vi "Test Step Stability.vi"(8 "Ranges":dbl[](array[numeric]), 9 "Setpoints":dbl[](array[numeric]), 11 "Array":refnum<class "TimeBasedQueue.lvclass">[](array[class])) -> (0 "Min":dbl[](array[numeric]), 1 "Components Stable?":bool[](array[boolean]), 2 "Max":dbl[](array[numeric]), 3 "System Stable?":bool)   [LabVIEW 2012, in "TimeBasedQueue.lvclass"]
uses:
  Time Based Queue/TimeBasedQueue.lvclass
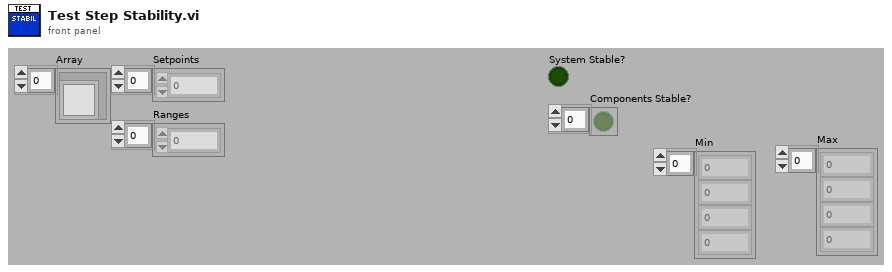
[diagram p1: front panel]
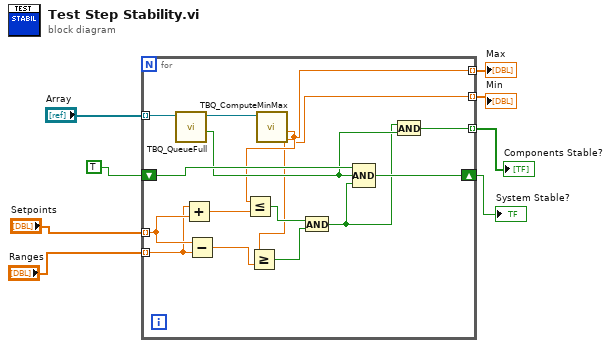
[diagram p0: block diagram]
diagram:
  n1 = for {
    tunnel: "Array" -> [w23] mode=indexing
    tunnel: "Setpoints" -> [w21] mode=indexing
    tunnel: "Ranges" -> [w20] mode=indexing
    shift-right: [w15] -> w4
    shift-left: TRUE ("x") -> [w14]
    tunnel: [w12] -> w3 mode=indexing
    tunnel: [w10] -> w2 mode=indexing
    tunnel: [w9] -> w1 mode=indexing
    n2 = call "TBQ_QueueFull.vi"("TBQ In"=w23) -> ("Queue Full?"=w13:bool, "TBQ Out"=w22:refnum<class "TimeBasedQueue.lvclass">)  [unwired: 9 in]
    n3 = Add(x=w20, y=w21) -> (x+y=w18:dbl)
    n4 = Subtract(x=w21, y=w20) -> (x-y=w19:dbl)
    n5 = call "TBQ_ComputeMinMax.vi"("TimeBasedQueue In"=w22) -> ("Minimum"=w9:dbl, "Maximum"=w10:dbl)  [unwired: 8 in, 1 out]
    n6 = Less Or Equal?(x=w10, y=w18) -> (x <= y?=w17:bool)
    n7 = Greater Or Equal?(x=w9, y=w19) -> (x >= y?=w16:bool)
    n8 = And(x=w17, y=w16) -> (x .and. y?=w11:bool)
    n9 = Compound Arithmetic op=AND(w14, w13, w11) -> (w15:bool)
    n10 = And(x=w11, y=w13) -> (x .and. y?=w12:bool)
  }
  "System Stable?" <- w4
  "Components Stable?" <- w3
  "Max" <- w2
  "Min" <- w1
